vi "Host Key.vi"(8 "Error In":errorcluster, 11 "Session In":refnum<class "Session.lvclass">) -> (0 "Error Out":errorcluster, 1 "Type":T1=1 items=["Unknown", "RSA", "DSS"], 2 "Host Key":u8[](array[numeric]), 3 "Sesssion Out":refnum<class "Session.lvclass">)   [LabVIEW 2021, in "Field_RnD_Services_LIBSSH2_Toolkit.lvlib" / "Session.lvclass"]
doc: "Gets the remote SSH server's host key."
uses:
  Session.lvclass
  Field_RnD_Services_LIBSSH2_Toolkit.lvlib
  SSH/SSH.lvclass
  Type Definitions/Host Key Types.ctl
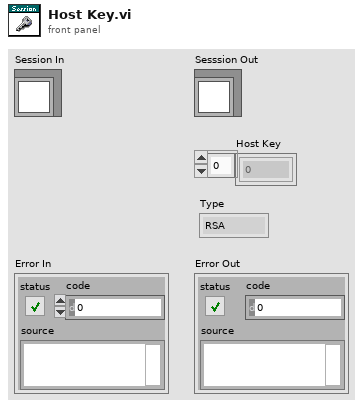
[diagram p1: front panel]
types:
  T1 = typedef "Field_RnD_Services_LIBSSH2_Toolkit.lvlib/Session.lvclass/Host Key Types.ctl" = i32
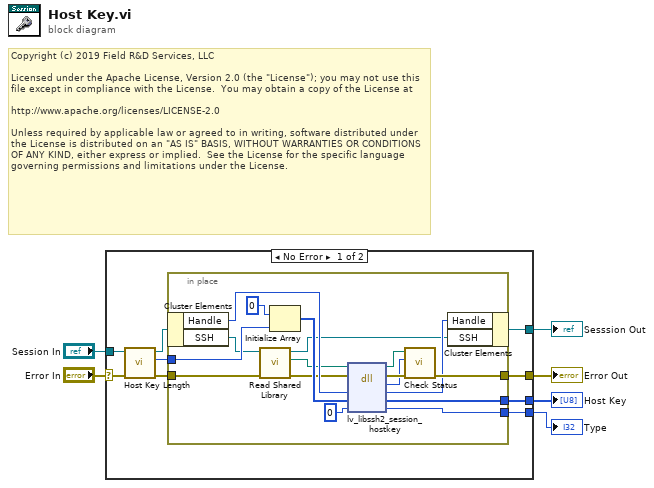
[diagram p0: block diagram]
diagram:
  # "Copyright (c) 2019 Field R&D Services, LLC\n\nLicensed under the Apache License, Version 2.0 (the \"License\"); you may not use this file except in compliance with the License.  You may obtain a copy of the License at\n\nhttp://www.apache.org/licenses/LICENSE-2.0\n\nUnless required by applicable law or agreed to in writing, software distributed under the License is distributed on an \"AS IS\" BASIS, WITHOUT WARRANTIES OR CONDITIONS OF ANY KIND, either express or implied.  See the License for the specific language governing permissions and limitations under the License."
  n1 = case shown="No Error" "Error In" {
    selector: "Error In" -> [w11 w34]
    tunnel: [w14 w34] -> w5
    tunnel: "Session In" -> [w13 w33]
    tunnel: [w15 w33] -> w3
    tunnel: [w8 _] -> w2
    tunnel: [w7 _] -> w1
    frame No Error {
      n2 = call "Host Key Length.vi"("Error In"=w11, "Session In"=w13) -> ("Error Out"=w10:errorcluster, "Length"=w9:i32, "Sesssion Out"=w12:refnum<class "Session.lvclass">)  [unwired: 7 in]
      n3 = in-place {
        in-place-border: [w30] -> w14
        in-place-border: w10 -> [w23]
        in-place-border: w9 -> [w24]
        in-place-border: [w21] -> w8
        in-place-border: [w16] -> w7
        n4 = in-place-cluster #1(w12) -> ("Handle"=w29:u64, "SSH"=w19:refnum<class "SSH.lvclass">)
        n5 = call "Read Shared Library.vi"("Error In"=w23, "SSH In"=w19) -> ("Error Out"=w20:errorcluster, "libssh2lv Shared Library"=w17:path, "SSH Out"=w18:refnum<class "SSH.lvclass">)  [unwired: 7 in]
        n6 = Initialize Array(u8 0, w24) -> (w26:u8[])
        n7 = dll-call lib="D:/Users/cfield/Code/Field R&D Services/SSH/LV-LIBSSH2/LabVIEW/trunk/src/Toolkit/Support/lv-libssh2.*" fn="lv_libssh2_session_hostkey"(path in=w17, error in=w20, "session"=w29, "buffer"=w26, "type"=0) -> (path out=w32:path, error out=w31:errorcluster, "result"=w25:i32, "session"=w28:u64, "buffer"=w21:u8[], "type"=w16:i32)  [unwired: 1 in]
        n8 = call "Check Status.vi"("Error In"=w31, "Status"=w25, "libssh2lv Shared Library In"=w32) -> ("Error Out"=w30:errorcluster)  [unwired: 7 in, 1 out]
        n9 = in-place-cluster #1("Handle"=w28, "SSH"=w18) -> (w15:refnum<class "Session.lvclass">)
      }
    }
    frame Error {
    }
  }
  "Sesssion Out" <- w3
  "Error Out" <- w5
  "Type" <- w1
  "Host Key" <- w2
